vi "START4LVADSPEEDPAUSE.vi"() -> ()   [LabVIEW 2024]
uses:
  <vilib>/Utility/file.llb/Read Delimited Spreadsheet (DBL).vi
  <vilib>/Instr/_visa.llb/VISA Configure Serial Port (Instr).vi
panel:
  out "THIS IS TO SEE THE STRING FROM SERIAL COMM PORT (TEMPORARY)":string
  out "LVAD Speed Waveform":dbl(graph)
  out "Flow Rate Waveform":dbl[](graph)
  in  "stop":bool
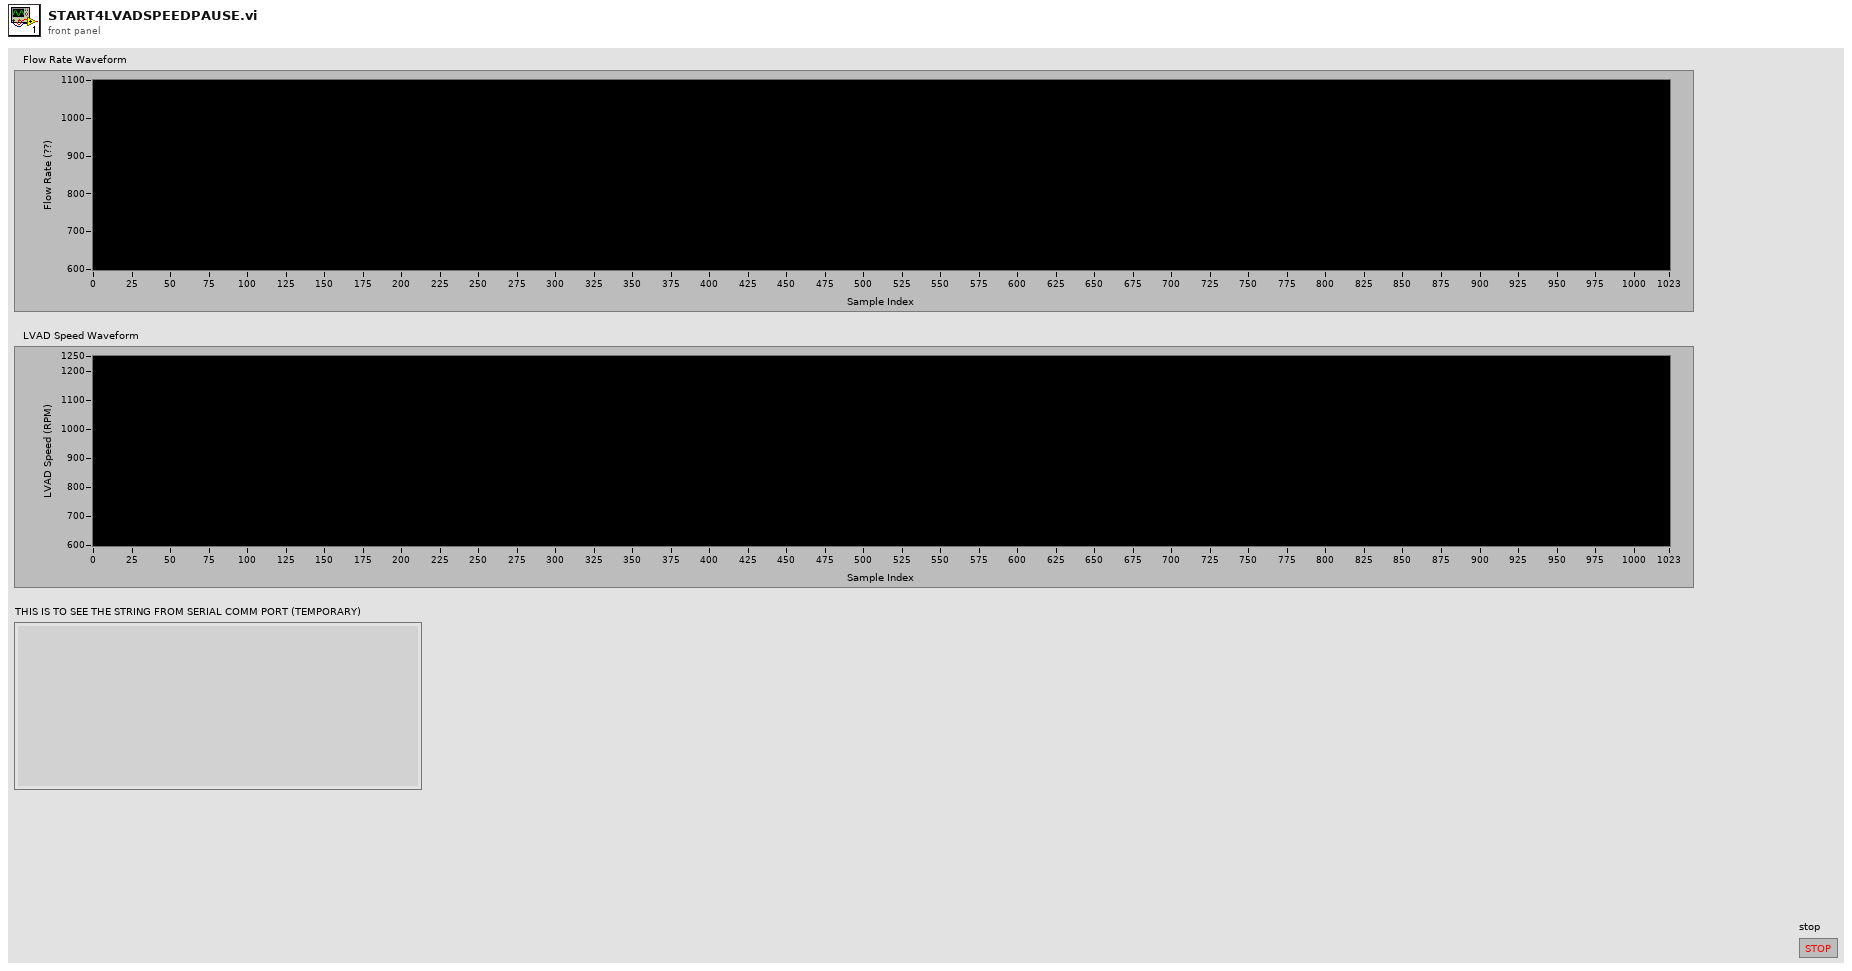
[diagram p1: front panel]
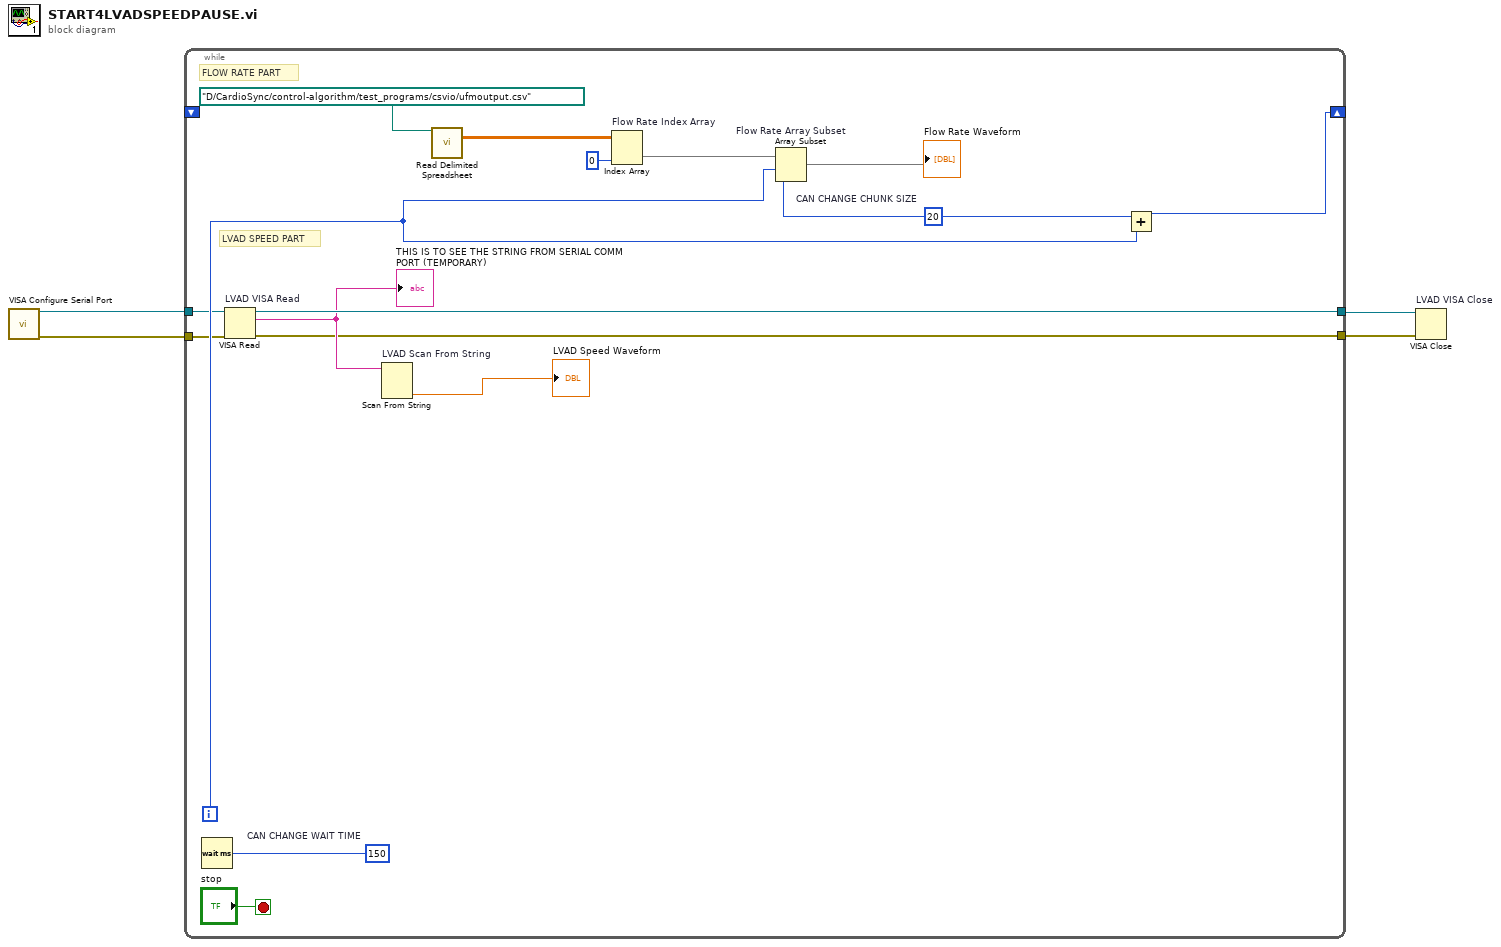
[diagram p0: block diagram]
diagram:
  n1 = call-poly "VISA Configure Serial Port"() -> ("VISA resource name out"=w4:refnum<visa-resource-name>, "error out"=w2:errorcluster)  [unwired: 14 in]
  n2 = while {
    shift-right: [w15] -> _
    shift-left: _ -> [_]
    tunnel: w4 -> [w10]
    tunnel: [w9] -> w3
    tunnel: w2 -> [w7]
    tunnel: [w6] -> w1
    i -> [w12]
    stop <- "stop" stop-if-true
    w16 = u32 150  # CAN CHANGE WAIT TIME
    w13 = 20  # CAN CHANGE CHUNK SIZE
    # "LVAD SPEED PART"
    # "FLOW RATE PART"
    n3 = Wait (ms)(milliseconds to wait=w16) -> ()  [unwired: 1 out]
    n4 = VISA Read "LVAD VISA Read"(VISA resource name=w10, error in (no error)=w7) -> (VISA resource name out=w9:refnum<visa-resource-name>, read buffer=w8:string, error out=w6:errorcluster)  [unwired: 1 in, 1 out]
    "THIS IS TO SEE THE STRING FROM SERIAL COMM PORT (TEMPORARY)" <- w8
    n5 = Scan From String "LVAD Scan From String"(input string=w8) -> (output 1=→"LVAD Speed Waveform":dbl)  [unwired: 4 in, 3 out]
    n6 = call-poly <vilib>:"Read Delimited Spreadsheet.vi"("file path (dialog if empty)"=path "D:/CardioSync/control-algorithm/test_programs/csvio/ufmoutput.csv") -> ("all rows"=w18:dbl[][])  [unwired: 9 in, 5 out]
    n7 = Index Array "Flow Rate Index Array"(array=w18, index (col)=0 ("disabled index (col)")) -> (element=w17:dbl[])  [unwired: 1 in]
    n8 = Array Subset "Flow Rate Array Subset"(array=w17, index=w12, length=w13) -> (→"Flow Rate Waveform":dbl[])
    n9 = Add(x=w13, y=w12) -> (x+y=w15:i32)
  }
  n10 = VISA Close "LVAD VISA Close"(VISA resource name=w3, error in (no error)=w1) -> ()  [unwired: 1 out]
